vi "12_Eoff.vi"(0 "file path (IN)":path, 1 "VGE":dbl, 5 "Project #":string, 7 "Request #":string, 9 "TEST #":string, 11 "error in (no error)":errorcluster) -> (4 "file path (OUT)":path, 6 "Eoff (uj)":dbl, 8 "DONE Eoff":bool, 10 "OFF Region":waveform(dbl)[](graph) caption="Eoff (uj)", 15 "error out":errorcluster)   [LabVIEW 2020]
uses:
  <vilib>/Waveform/WDTOps.llb/WDT Waveform Duration DBL.vi
  <vilib>/Waveform/WDTOps.llb/WDT Get Waveform Subset DBL.vi
  <vilib>/measure/mamon.llb/Trigger Detection for 1 Channel.vi
  <vilib>/measure/mascope.llb/Transition Measurements 1 chan.vi
  <vilib>/measure/NI_MAPro.lvlib
panel:
  in  "Decision ?":bool
  out "Cursor a : Channel 2":dbl
  in  "Cursor a : Channel 2\nfall edge tolerance":dbl=0.1
  in  "Cursor a : Channel 2\nfall edge number":i32=1 min=1
  out "Eoff : XY Graph":cluster{"X":dbl, "Y":dbl}[](graph)
  out "Eoff Area Y-axis":dbl[](array[numeric])
  out "Eoff Area X-axis":dbl[](array[numeric])
  out "90% Vge":dbl
  out "measurement info (CH2)":T1 {"ref levels"."ref units" items=["absolute", "relative"]; "ref levels"."high ref level" format="%.2p"; "ref levels"."low ref level" format="%.2p"; "ref levels"."mid ref level" format="%.2p"; "end time" format="%.6e"; "start time" format="%.6e"}
  in  "reference  levels (CH2 initialize)":T2={"high ref level"=90.0, "mid ref level"=50.0, "low ref level"=10.0, "ref units"=1} {"ref units" items=["absolute", "percent"]; "high ref level" format="%0.2f"; "low ref level" format="%0.2f"; "mid ref level" format="%0.2f"}
  out "Waveform Graph":waveform(dbl)[](graph)
  # "From 90% Vge to Most Right of Screen"
  # "Default = 1"
  # "Default = 0.1"
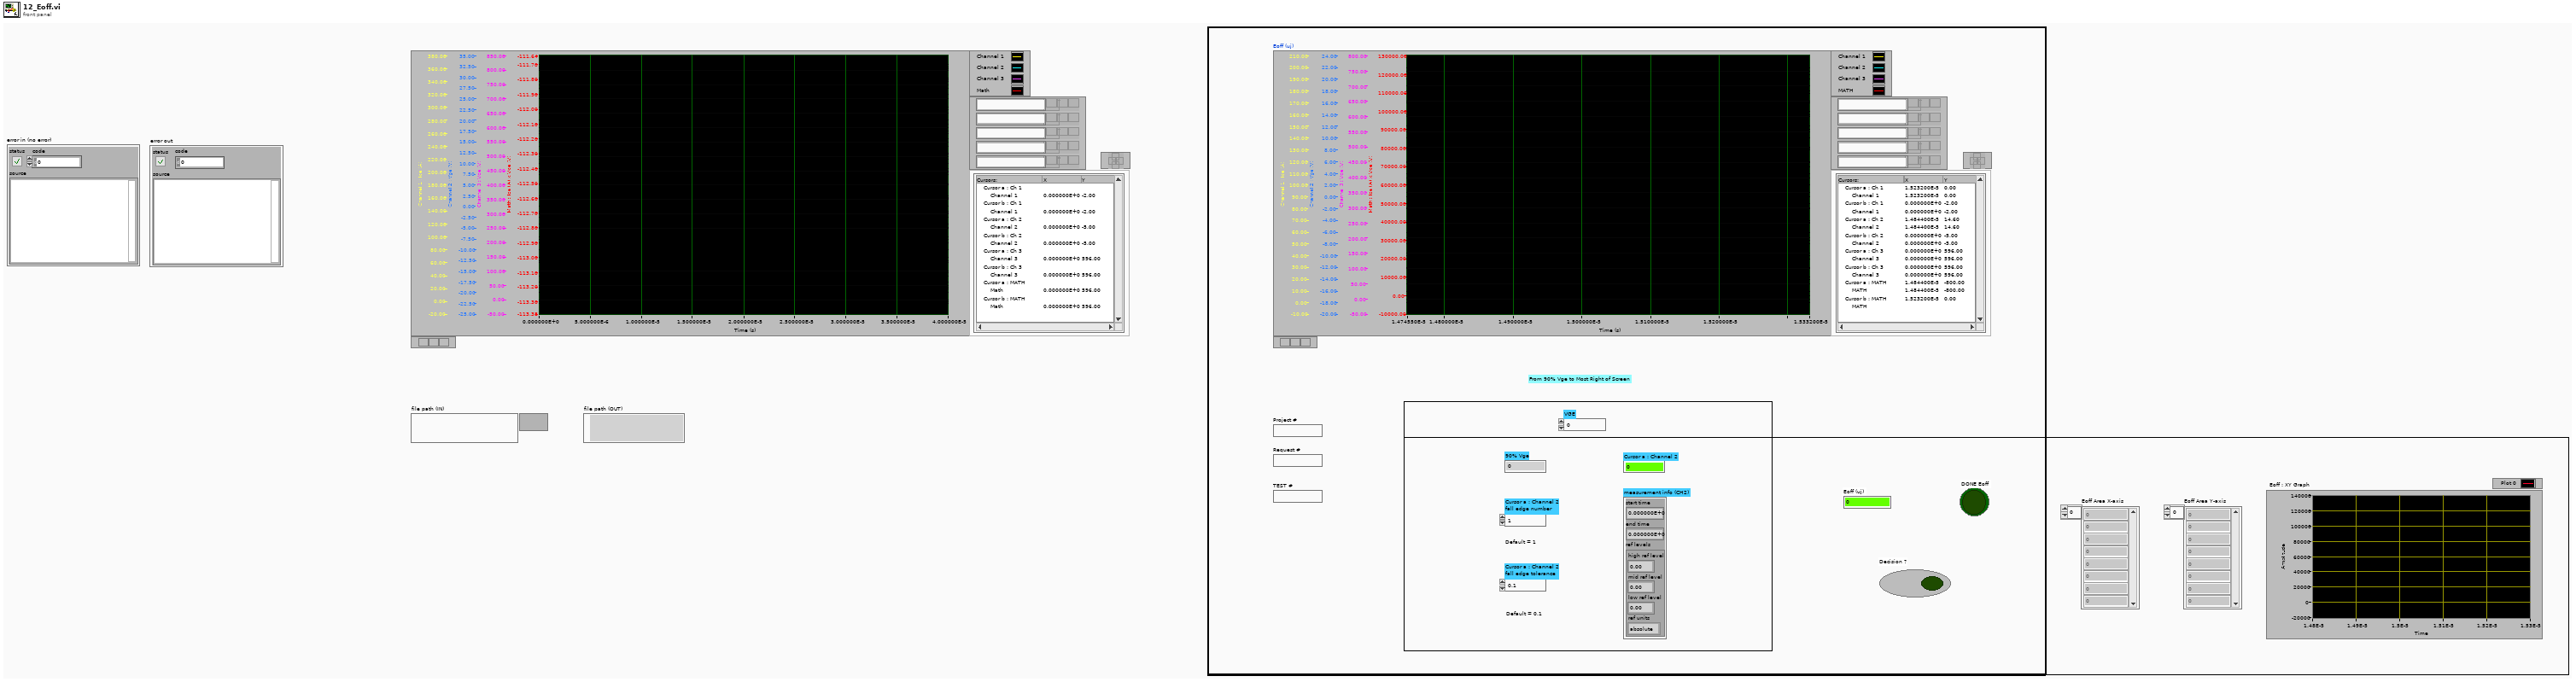
[diagram p1: front panel]
types:
  T1 = cluster{"start time":dbl, "end time":dbl, "ref levels":cluster{"high ref level":dbl, "mid ref level":dbl, "low ref level":dbl, "ref units":u16}}
  T2 = cluster{"high ref level":dbl, "mid ref level":dbl, "low ref level":dbl, "ref units":u16}
  T3 = enum32{"Invalid", "Standard", "Closed", "Hidden", "Minimized", "Maximized"}
  T4 = typedef "imagedata.ctl" = cluster{"image type":i32, "image depth":i32, "image":u8[], "mask":u8[], "colors":u32[], "Rectangle":cluster{"left":i16, "top":i16, "right":i16, "bottom":i16}}
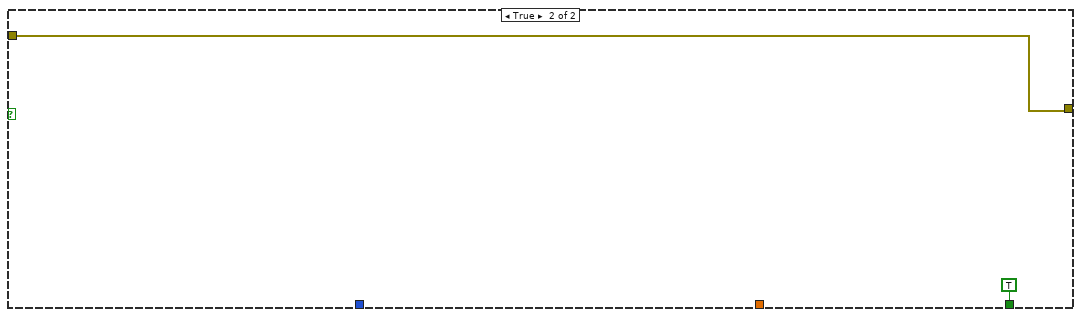
[diagram p8: hidden frame]
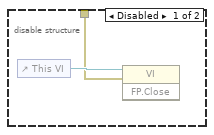
[diagram p9: hidden frame]
diagram:
  w10 = 0.0 ("Eoff (uj)")
  w14 = errorcluster {"status"=FALSE, "code"=0, "source"=""} ("error out")
  w3 = FALSE ("DONE Tdon")
  w15 = waveform(dbl)[] [] ("Waveform Graph")
  n1 = local write "error out"(w14) -> ()
  n2 = local write "error in (no error)"(w14) -> ()
  n3 = local write "Cursor a : Channel 2\nfall edge tolerance"(0.1 ("Cursor a : Channel 2\nfall edge tolerance")) -> ()
  n4 = local write "Cursor a : Channel 2\nfall edge number"(1 ("Cursor a : Channel 2\nfall edge number")) -> ()
  n5 = local write "DONE Eoff"(w3) -> ()
  n6 = local write "Decision ?"(w3) -> ()
  n7 = local write "Eoff (uj)"(w10) -> ()
  n8 = local write "Cursor a : Channel 2"(w10) -> ()
  n9 = local write "Waveform Graph"(w15) -> ()
  n10 = local write "OFF Region"(w15) -> ()
  n11 = flat-sequence {
    tunnel: [w17] -> w5
    tunnel: ["file path (IN)"] -> w4
    tunnel: [w27] -> w9
    tunnel: [w26] -> w7
    tunnel: w5 -> [w25]
    tunnel: w4 -> [w24]
    tunnel: w9 -> [w376]
    tunnel: [w375] -> w8
    tunnel: w7 -> [w374]
    tunnel: [w374] -> w6
    tunnel: w8 -> [w389]
    tunnel: w6 -> [w390]
    frame #0 {
      n12 = control-ref of="This VI"() -> (w19:refnum<vi>)
      n13 = invoke class="VI" method="FP.Open"(reference=w19, error in="error in (no error)", "Activate"=TRUE ("Activate?"), "State"=T3."Maximized") -> (error out=w20:errorcluster)  [unwired: 1 in, 4 out]
      n14 = property class="VI"(reference=w19, error in=w20, "Front Panel.Closeable"=TRUE ("Front Panel Window:Closeable")) -> (error out=w17:errorcluster)  [unwired: 1 out]
    }
    frame #1 {
      n15 = while {
        shift-right: [w33] -> w27
        shift-left: w25 -> [w35]
        tunnel: [w30] -> w26
        tunnel: w24 -> [w29]
        stop <- w31 stop-if-true
        n16 = flat-sequence {
          tunnel: [w70] -> w62
          tunnel: w35 -> [w76]
          tunnel: [w76] -> w34
          tunnel: w29 -> [w70]
          tunnel: w62 -> [w178]
          tunnel: [w110] -> w61
          tunnel: [w109] -> w60
          tunnel: [w99] -> w59
          tunnel: [w81] -> w58
          tunnel: [w79] -> w57
          tunnel: w34 -> [w183]
          tunnel: [w77] -> w28
          tunnel: w61 -> [w208]
          tunnel: w60 -> [w201]
          tunnel: [w213] -> w56
          tunnel: w59 -> [w212]
          tunnel: [w212] -> w55
          tunnel: [w199] -> w54
          tunnel: [w205] -> w53
          tunnel: w58 -> [w209]
          tunnel: [w209] -> w52
          tunnel: w57 -> [w206]
          tunnel: w28 -> [w200]
          tunnel: w56 -> [w250]
          tunnel: [w249] -> w51
          tunnel: w55 -> [w255]
          tunnel: [w255] -> w50
          tunnel: w54 -> [w254]
          tunnel: [w254] -> w49
          tunnel: w53 -> [w253]
          tunnel: [w253] -> w48
          tunnel: w52 -> [w252]
          tunnel: [w252] -> w47
          tunnel: w51 -> [w266]
          tunnel: [w257] -> w46
          tunnel: w50 -> [w267]
          tunnel: [w267] -> w45
          tunnel: w49 -> [w265]
          tunnel: [w265] -> w44
          tunnel: w48 -> [w264]
          tunnel: [w264] -> w43
          tunnel: w47 -> [w262]
          tunnel: w46 -> [w348]
          tunnel: [w347] -> w42
          tunnel: w45 -> [w355]
          tunnel: [w355] -> w41
          tunnel: w44 -> [w344]
          tunnel: w43 -> [w343]
          tunnel: [w343] -> w40
          tunnel: [w344] -> w39
          tunnel: w42 -> [w365]
          tunnel: [w366] -> w38
          tunnel: w41 -> [w367]
          tunnel: [w367] -> w37
          tunnel: w40 -> [w360]
          tunnel: w39 -> [w359]
          tunnel: w38 -> [w370]
          tunnel: w37 -> [w368]
          tunnel: [w369] -> w36
          tunnel: [w368] -> w30
          frame #0 {
            w69 = FALSE ("DONE Tdon")
            w75 = waveform(dbl)[] [] ("Waveform Graph")
            w74 = 0.0 ("Eoff (uj)")
            n17 = local write "DONE Eoff"(w69) -> ()
            n18 = local write "Decision ?"(w69) -> ()
            n19 = local write "Eoff (uj)"(w74) -> ()
            n20 = local write "Cursor a : Channel 2"(w74) -> ()
            n21 = local write "Waveform Graph"(w75) -> ()
            n22 = local write "OFF Region"(w75) -> ()
            n23 = local write "Eoff Area Y-axis"(dbl[] [] ("Eoff Area X-axis")) -> ()
            n24 = local write "Eoff Area X-axis"(dbl[] [] ("Eoff Area Y-axis")) -> ()
            n25 = local write "Eoff : XY Graph"(cluster{"X":dbl, "Y":dbl}[] [] ("Eoff : XY Graph")) -> ()
          }
          frame #1 {
            w78 = 0.0 ("start samples/time")
            w88 = u16 1 items=["Samples", "Relative Time"] ("start/duration format")
            w160 = u16 1 items=["Samples", "Relative Time"] ("start/duration format")
            w170 = u16 1 items=["Samples", "Relative Time"] ("start/duration format")
            w171 = u16 1 items=["Samples", "Relative Time"] ("start/duration format")
            # "Channel 3"
            # "Channel 1"
            # "Channel MATH"
            # "MATH = Ch1 x Ch3"
            # "Channel 1"
            # "Channel 3"
            # "Channel 2"
            # "dt"
            # "Ch2"
            # "Ch1"
            n26 = call "3_ReadDatatoWaveform.vi"("error in (no error)"=w183, "file path (IN)"=w178) -> ("error out"=w157:errorcluster, "Waveform Graph"=→"Waveform Graph":waveform(dbl)[], "file path (OUT)"=w99:path, "dt"=w179:dbl, "Ch 2 Data"=w176:dbl[], "Ch 3 Data"=w180:dbl[], "Ch 1 Data"=w177:dbl[])  [unwired: 3 in]
            n27 = call <vilib>:"Beep.vi"("use system alert? (T)"=FALSE, "duration (msec)"=u32 200, "frequency (Hz)"=u32 2000) -> ()  [unwired: 9 in]
            n28 = To Time Stamp(1:0.0 ("number")) -> (0:w181:timestamp)
            n29 = disable-structure shown="Enabled" {
              disable-tunnel: w181 -> [w198 _]
              disable-tunnel: w179 -> [w197 _]
              disable-tunnel: w180 -> [w196 _]
              disable-tunnel: [w195 _] -> w95
              frame Enabled {
                # "Channel 3"
                n30 = Bundle By Name("Y"=w196, "dt"=w197, "t0"=w198) -> (w195:waveform(dbl))  [unwired: 1 in]
              }
              frame Disabled {
              }
            }
            n31 = disable-structure shown="Enabled" {
              disable-tunnel: w181 -> [w194 _]
              disable-tunnel: w179 -> [w193 _]
              disable-tunnel: w176 -> [w192 _]
              disable-tunnel: [w191 _] -> w159
              frame Enabled {
                # "Channel 2"
                n32 = Bundle By Name("Y"=w192, "dt"=w193, "t0"=w194) -> (w191:waveform(dbl))  [unwired: 1 in]
              }
              frame Disabled {
              }
            }
            n33 = disable-structure shown="Enabled" {
              disable-tunnel: w181 -> [w190 _]
              disable-tunnel: w179 -> [w189 _]
              disable-tunnel: w177 -> [w188 _]
              disable-tunnel: [w187 _] -> w96
              frame Enabled {
                # "Channel 1"
                n34 = Bundle By Name("Y"=w188, "dt"=w189, "t0"=w190) -> (w187:waveform(dbl))  [unwired: 1 in]
              }
              frame Disabled {
              }
            }
            n35 = Unbundle By Name(w95) -> ("Y"=w92:dbl[])
            n36 = Unbundle By Name(w96) -> ("Y"=w93:dbl[], "dt"=w80:dbl, "t0"=w94:timestamp)
            n37 = for {
              tunnel: w93 -> [w186] mode=indexing
              tunnel: w92 -> [w185] mode=indexing
              tunnel: [w184] -> w91 mode=indexing
              n38 = Multiply(x=w186, y=w185) -> (x*y=w184:dbl)
            }
            n39 = Bundle By Name("Y"=w91, "dt"=w80, "t0"=w94) -> (w83:waveform(dbl))  [unwired: 1 in]
            n40 = call-poly <vilib>:"Waveform Duration.vi"("waveform in"=w83) -> ("error out"=w84:errorcluster, "duration"=w86:dbl, "waveform out"=w89:waveform(dbl))  [unwired: 8 in]
            n41 = call-poly <vilib>:"Waveform Duration.vi"("error in (no error)"=w157, "waveform in"=w95) -> ("error out"=w164:errorcluster, "duration"=w162:dbl, "waveform out"=w97:waveform(dbl))  [unwired: 7 in]
            n42 = call-poly <vilib>:"Waveform Duration.vi"("error in (no error)"=w157, "waveform in"=w159) -> ("error out"=w165:errorcluster, "duration"=w168:dbl, "waveform out"=w166:waveform(dbl))  [unwired: 7 in]
            n43 = call-poly <vilib>:"Waveform Duration.vi"("error in (no error)"=w157, "waveform in"=w96) -> ("error out"=w175:errorcluster, "duration"=w172:dbl, "waveform out"=w174:waveform(dbl))  [unwired: 7 in]
            n44 = Divide(x=w86, y=2.0) -> (x/y=w87:dbl)
            n45 = Divide(x=w162, y=2.0) -> (x/y=w161:dbl)
            n46 = Divide(x=w168, y=2.0) -> (x/y=w169:dbl)
            n47 = Divide(x=w172, y=2.0) -> (x/y=w79:dbl)
            n48 = call-poly <vilib>:"Get Waveform Subset.vi"("start/duration format"=w160, "error in (no error)"=w164, "duration"=w161, "start samples/time"=w78, "waveform in"=w97) -> ("error out"=w154:errorcluster, "waveform out"=w98:waveform(dbl))  [unwired: 1 in, 2 out]
            n49 = call-poly <vilib>:"Get Waveform Subset.vi"("start/duration format"=w88, "error in (no error)"=w84, "duration"=w87, "start samples/time"=w78, "waveform in"=w89) -> ("error out"=w82:errorcluster, "waveform out"=w81:waveform(dbl))  [unwired: 1 in, 2 out]
            n50 = call-poly <vilib>:"Get Waveform Subset.vi"("start/duration format"=w170, "error in (no error)"=w165, "duration"=w169, "start samples/time"=w78, "waveform in"=w166) -> ("error out"=w155:errorcluster, "waveform out"=w110:waveform(dbl))  [unwired: 1 in, 2 out]
            n51 = call-poly <vilib>:"Get Waveform Subset.vi"("start/duration format"=w171, "error in (no error)"=w175, "duration"=w79, "start samples/time"=w78, "waveform in"=w174) -> ("error out"=w156:errorcluster, "waveform out"=w77:waveform(dbl))  [unwired: 1 in, 2 out]
            n52 = Build Array(w77, w110, w98, w81) -> (→"OFF Region":waveform(dbl)[])
            n53 = Merge Errors(w156, w155, w154, w82) -> (w107:errorcluster)
            n54 = property on="OFF Region" class="WFGraph (strict)"(error in=w107) -> (error out=w106:errorcluster, "Width"=w105:u32)  [unwired: 1 in, 1 out]
            n55 = property on="OFF Region" class="WFGraph (strict)"(error in=w106, "Caption.Justify"=enum16{"Left", "Center", "Right"}."Left" ("Caption.Justification"), "Caption.Width"=w105, "Caption.FontBold"=TRUE ("Caption.Font:Bold"), "Caption.FontColor"=u32 16860 ("Caption.Font:Color"), "Caption.FontSize"=u32 24 ("Caption.Font:Size"), "Caption.Text"="Eoff (uj)") -> (error out=w101:errorcluster)  [unwired: 1 in, 1 out]
            n56 = property on="OFF Region" class="WFGraph (strict)"(error in=w101, "XScale.Offset"=w78) -> (error out=w134:errorcluster)  [unwired: 1 in, 1 out]
            n57 = property on="OFF Region" class="WFGraph (strict)"(error in=w134, "Active Cursor"=u32 0, "Cursor.Cursor X"=0.0 ("Cursor.Cursor Position:Cursor X"), "Cursor.Cursor Y"=0.0 ("Cursor.Cursor Position:Cursor Y"), "Cursor.Visible"=FALSE) -> (error out=w133:errorcluster)  [unwired: 1 in, 1 out]
            n58 = property on="OFF Region" class="WFGraph (strict)"(error in=w133, "Active Cursor"=u32 1, "Cursor.Cursor X"=0.0 ("Cursor.Cursor Position:Cursor X"), "Cursor.Cursor Y"=0.0 ("Cursor.Cursor Position:Cursor Y"), "Cursor.Visible"=FALSE) -> (error out=w132:errorcluster)  [unwired: 1 in, 1 out]
            n59 = property on="OFF Region" class="WFGraph (strict)"(error in=w132, "Active Cursor"=u32 2, "Cursor.Cursor X"=0.0 ("Cursor.Cursor Position:Cursor X"), "Cursor.Cursor Y"=0.0 ("Cursor.Cursor Position:Cursor Y"), "Cursor.Visible"=FALSE) -> (error out=w131:errorcluster)  [unwired: 1 in, 1 out]
            n60 = property on="OFF Region" class="WFGraph (strict)"(error in=w131, "Active Cursor"=u32 3, "Cursor.Cursor X"=0.0 ("Cursor.Cursor Position:Cursor X"), "Cursor.Cursor Y"=0.0 ("Cursor.Cursor Position:Cursor Y"), "Cursor.Visible"=FALSE) -> (error out=w114:errorcluster)  [unwired: 1 in, 1 out]
            n61 = property on="OFF Region" class="WFGraph (strict)"(error in=w114, "Active Cursor"=u32 4, "Cursor.Cursor X"=0.0 ("Cursor.Cursor Position:Cursor X"), "Cursor.Cursor Y"=0.0 ("Cursor.Cursor Position:Cursor Y"), "Cursor.Visible"=FALSE) -> (error out=w113:errorcluster)  [unwired: 1 in, 1 out]
            n62 = property on="OFF Region" class="WFGraph (strict)"(error in=w113, "Active Cursor"=u32 5, "Cursor.Cursor X"=0.0 ("Cursor.Cursor Position:Cursor X"), "Cursor.Cursor Y"=0.0 ("Cursor.Cursor Position:Cursor Y"), "Cursor.Visible"=FALSE) -> (error out=w112:errorcluster)  [unwired: 1 in, 1 out]
            n63 = property on="OFF Region" class="WFGraph (strict)"(error in=w112, "Active Cursor"=u32 6, "Cursor.Cursor X"=0.0 ("Cursor.Cursor Position:Cursor X"), "Cursor.Cursor Y"=0.0 ("Cursor.Cursor Position:Cursor Y"), "Cursor.Visible"=FALSE) -> (error out=w111:errorcluster)  [unwired: 1 in, 1 out]
            n64 = property on="OFF Region" class="WFGraph (strict)"(error in=w111, "Active Cursor"=u32 7, "Cursor.Cursor X"=0.0 ("Cursor.Cursor Position:Cursor X"), "Cursor.Cursor Y"=0.0 ("Cursor.Cursor Position:Cursor Y"), "Cursor.Visible"=FALSE) -> (error out=w109:errorcluster)  [unwired: 1 in, 1 out]
          }
          frame #2 {
            w230 = u16 0 items=["falling", "rising"] ("polarity (rising)")
            # "Cursor a : Channel 1"
            # "Channel 1"
            # "2nd PARAMETER"
            # "MOST RIGHT SCREEN"
            # "Cursor a : Channel 2"
            # "End Time 1st Cursor"
            # "2nd PARAMETER"
            # "MOST RIGHT SCREEN"
            # "1st PARAMETER"
            # "Channel 2"
            n65 = Divide(x=90.0, y=100.0) -> (x/y=w234:dbl)
            n66 = Multiply(x=w234, y="VGE") -> (x*y=w207:dbl)
            "90% Vge" <- w207
            n67 = Add(x=w207, y="Cursor a : Channel 2\nfall edge tolerance") -> (x+y=w229:dbl)
            n68 = Subtract(x=w207, y="Cursor a : Channel 2\nfall edge tolerance") -> (x-y=w228:dbl)
            n69 = Bundle By Name(cluster="reference  levels (CH2 initialize)", "high ref level"=w229, "mid ref level"=w207, "low ref level"=w228, "ref units"=u16 0) -> (w225:T2)
            n70 = call-poly <vilib>:"Transition Measurements.vi"("edge number (1)"="Cursor a : Channel 2\nfall edge number", "error in (no error)"=w201, "reference levels"=w225, "polarity (rising)"=w230, "signal in"=w208) -> ("error out"=w219:errorcluster, "measurement info"=w224:T1)  [unwired: 1 in, 4 out]
            "measurement info (CH2)" <- w224
            n71 = disable-structure shown="Enabled" {
              disable-tunnel: [w245 _] -> w202
              disable-tunnel: w201 -> [w244 _]
              disable-tunnel: w200 -> [w243 _]
              disable-tunnel: [w241 _] -> w199
              frame Enabled {
                w247 = u16 0 items=["Falling Edge", "Rising Edge"] ("trigger slope")
                w246 = u16 1 items=["Index", "Time"] ("location mode")
                n72 = call-poly <vilib>:"Basic Level Trigger Detection.vi"("signal in"=w243, "level"=0.2, "hysteresis"=10.0, "location mode"=w246, "error in (no error)"=w244, "trigger slope"=w247) -> ("trigger location"=w241:dbl, "error out"=w245:errorcluster)  [unwired: 7 in, 1 out]
              }
              frame Disabled {
              }
            }
            n73 = Unbundle By Name(w224) -> ("end time"=w205:dbl)
            n74 = call <vilib>:"Beep.vi"("use system alert? (T)"=FALSE, "duration (msec)"=u32 200, "frequency (Hz)"=u32 2000) -> ()  [unwired: 9 in]
            n75 = disable-structure shown="Disabled" {
              disable-tunnel: w206 -> [w237 _]
              disable-tunnel: [w236 _] -> _
              disable-tunnel: w205 -> [w235 _]
              frame Disabled {
                n76 = Add(x=w237, y=w235) -> (x+y=w239:dbl)
                n77 = Divide(x=w239, y=2.0) -> (x/y=w236:dbl)
              }
              frame Enabled {
              }
            }
            n78 = disable-structure shown="Disabled" {
              frame Disabled {
                # "3"
                # "Cursor b : Channel 2"
              }
              frame Enabled {
              }
            }
            n79 = property on="OFF Region" class="WFGraph (strict)"(error in=w219, "Active Cursor"=u32 2, "Cursor.Cursor X"=w205, "Cursor.Visible"=TRUE, "Cursor.Cursor Name Visible"=TRUE) -> (error out=w214:errorcluster)  [unwired: 1 in, 1 out]
            n80 = property on="OFF Region" class="WFGraph (strict)"(error in=w202, "Active Cursor"=u32 0, "Cursor.Cursor X"=w199, "Cursor.Visible"=TRUE, "Cursor.Cursor Name Visible"=TRUE) -> (error out=w215:errorcluster)  [unwired: 1 in, 1 out]
            n81 = Merge Errors(w215, w214) -> (w213:errorcluster)
          }
          frame #3 {
            # "Cursor a : Channel 2"
            n82 = property on="OFF Region" class="WFGraph (strict)"(error in=w250, "Active Cursor"=u32 2) -> (error out=w249:errorcluster, "Cursor.Cursor Y"=→"Cursor a : Channel 2":dbl)  [unwired: 1 in, 1 out]
          }
          frame #4 {
            n83 = flat-sequence {
              tunnel: w266 -> [w271]
              tunnel: w265 -> [w273]
              tunnel: w264 -> [w272]
              tunnel: [w268] -> w263
              tunnel: w263 -> [w282]
              tunnel: w261 -> [w281]
              tunnel: [w280] -> w260
              tunnel: w260 -> [w323]
              tunnel: [w325] -> w259
              tunnel: [w324] -> w258
              tunnel: [w323] -> w256
              tunnel: w259 -> [w331]
              tunnel: w258 -> [w330]
              tunnel: [w329] -> w257
              tunnel: w256 -> [w329]
              frame #0 {
                # "Cursor a : MATH"
                # "Cursor b : MATH"
                n84 = property on="OFF Region" class="WFGraph (strict)"(error in=w271, "Active Cursor"=u32 7, "Cursor.Cursor X"=w273, "Cursor.Visible"=TRUE, "Cursor.Cursor Name Visible"=TRUE) -> (error out=w269:errorcluster)  [unwired: 1 in, 1 out]
                n85 = property on="OFF Region" class="WFGraph (strict)"(error in=w271, "Active Cursor"=u32 6, "Cursor.Cursor X"=w272, "Cursor.Visible"=TRUE, "Cursor.Cursor Name Visible"=TRUE) -> (error out=w270:errorcluster)  [unwired: 1 in, 1 out]
                n86 = Merge Errors(w269, w270) -> (w268:errorcluster)
              }
              frame #1 {
                n87 = while {
                  tunnel: w282 -> [w290]
                  tunnel: w281 -> [w284]
                  tunnel: [w283] -> w280
                  i -> [w285]
                  stop <- w288 stop-if-true
                  # "Cursor b : MATH"
                  # "Cursor a : MATH"
                  n88 = property on="OFF Region" class="WFGraph (strict)"(error in=w290, "Active Cursor"=u32 7) -> (error out=w294:errorcluster, "Cursor.Cursor X"=w296:dbl)  [unwired: 1 in, 1 out]
                  n89 = property on="OFF Region" class="WFGraph (strict)"(error in=w290, "Active Cursor"=u32 6) -> (error out=w293:errorcluster, "Cursor.Cursor X"=w295:dbl)  [unwired: 1 in, 1 out]
                  n90 = Merge Errors(w293, w294) -> (w286:errorcluster)
                  n91 = Equal?(x=w295, y=w296) -> (x = y?=w289:bool)
                  n92 = case shown="False" w289 {
                    tunnel: [FALSE TRUE] -> w288
                    tunnel: w286 -> [w301 w321]
                    tunnel: w285 -> [w300 _]
                    tunnel: w284 -> [w298 _]
                    tunnel: [w297 w321] -> w283
                    frame False {
                      n93 = flat-sequence {
                        tunnel: w301 -> [w311]
                        tunnel: w300 -> [w306]
                        tunnel: [w303] -> w299
                        tunnel: w299 -> [w316]
                        tunnel: w298 -> [w314]
                        tunnel: [w313] -> w297
                        frame #0 {
                          # "Cursor a : MATH"
                          n94 = property on="OFF Region" class="WFGraph (strict)"(error in=w311, "Active Cursor"=u32 6) -> (error out=w303:errorcluster, "Cursor.Cursor X"=w308:dbl, "Cursor.Cursor Y"=w307:dbl)  [unwired: 1 in, 1 out]
                          n95 = local read "Eoff Area Y-axis"() -> (w309:dbl[])
                          n96 = local read "Eoff Area X-axis"() -> (w310:dbl[])
                          n97 = Insert Into Array(array=w309, index=w306, new element=w307) -> (w304:dbl[])
                          n98 = Insert Into Array(array=w310, index=w306, new element=w308) -> (w305:dbl[])
                          n99 = local write "Eoff Area X-axis"(w305) -> ()
                          n100 = local write "Eoff Area Y-axis"(w304) -> ()
                        }
                        frame #1 {
                          # "Cursor a : MATH"
                          # "Cursor a : MATH"
                          n101 = property on="OFF Region" class="WFGraph (strict)"(error in=w316, "Active Cursor"=u32 6) -> (error out=w315:errorcluster, "Cursor.Cursor X"=w318:dbl)  [unwired: 1 in, 1 out]
                          n102 = Add(x=w318, y=w314) -> (x+y=w317:dbl)
                          n103 = property on="OFF Region" class="WFGraph (strict)"(error in=w315, "Active Cursor"=u32 6, "Cursor.Cursor X"=w317) -> (error out=w313:errorcluster)  [unwired: 1 in, 1 out]
                        }
                      }
                    }
                    frame True {
                    }
                  }
                  n104 = Wait (ms)(milliseconds to wait=u32 1) -> ()  [unwired: 1 out]
                }
              }
              frame #2 {
                n105 = local read "Eoff Area X-axis"() -> (w325:dbl[])
                n106 = local read "Eoff Area Y-axis"() -> (w324:dbl[])
                n107 = Build Cluster Array(w325, w324) -> (w326:cluster{dbl, dbl}[])
                n108 = local write "Eoff : XY Graph"(w326) -> ()
                n109 = Wait (ms)(milliseconds to wait=u32 50) -> ()  [unwired: 1 out]
              }
              frame #3 {
                n110 = Wait (ms)(milliseconds to wait=u32 50) -> ()  [unwired: 1 out]
                n111 = Delete From Array(array=w331, index=0) -> (array with subset deleted=w341:dbl[])  [unwired: 1 in, 1 out]
                n112 = Delete From Array(array=w330, index=0) -> (array with subset deleted=w335:dbl[])  [unwired: 1 in, 1 out]
                n113 = Subtract(x=w341, y=w331) -> (x-y=w340:dbl[])
                n114 = Add(x=w335, y=w330) -> (x+y=w339:dbl[])
                n115 = Compound Arithmetic op=MULTIPLY(w340, w339, invert 2.0 ("Numeric")) -> (w337:dbl[])
                n116 = Add Array Elements(numeric array=w337) -> (sum=w333:dbl)
                n117 = Multiply(x=w333, y=1000000.0) -> (x*y=→"Eoff (uj)":dbl)
              }
            }
            n118 = Unbundle By Name(w262) -> ("dt"=w261:dbl)
          }
          frame #5 {
            # "Cursor a : MATH"
            # "Cursor b : MATH"
            n119 = property on="OFF Region" class="WFGraph (strict)"(error in=w348, "Active Cursor"=u32 7, "Cursor.Cursor X"=w344, "Cursor.Visible"=TRUE, "Cursor.Cursor Name Visible"=TRUE) -> (error out=w345:errorcluster)  [unwired: 1 in, 1 out]
            n120 = property on="OFF Region" class="WFGraph (strict)"(error in=w348, "Active Cursor"=u32 6, "Cursor.Cursor X"=w343, "Cursor.Visible"=TRUE, "Cursor.Cursor Name Visible"=TRUE) -> (error out=w346:errorcluster)  [unwired: 1 in, 1 out]
            n121 = Merge Errors(w345, w346) -> (w347:errorcluster)
          }
          frame #6 {
            # "2nd Cursor"
            # "1st Cursor"
            n122 = Subtract(x=w360, y=1e-07) -> (x-y=w361:dbl)
            n123 = Add(x=w359, y=1e-07) -> (x+y=w362:dbl)
            n124 = call <vilib>:"Beep.vi"("use system alert? (T)"=FALSE, "duration (msec)"=u32 200, "frequency (Hz)"=u32 2000) -> ()  [unwired: 9 in]
            n125 = property on="OFF Region" class="WFGraph (strict)"(error in=w365, "XScale.Minimum"=w361, "XScale.Maximum"=w362) -> (error out=w366:errorcluster)  [unwired: 1 in, 1 out]
          }
          frame #7 {
            n126 = while {
              shift-right: [w371] -> w369
              shift-left: w370 -> [w371]
              stop <- "Decision ?" stop-if-true
              n127 = Wait (ms)(milliseconds to wait=u32 100) -> ()  [unwired: 1 out]
            }
          }
        }
        n128 = while {
          tunnel: [w64] -> w31
          shift-right: [w67] -> w33
          shift-left: w36 -> [w68]
          stop <- w66 stop-if-true
          n129 = Wait (ms)(milliseconds to wait=u32 100) -> ()  [unwired: 1 out]
          n130 = call "Display Message to User"("error in (no error)"=w68) -> ("error out"=w67:errorcluster, "NO"=w64:bool)  [unwired: 9 in]
          n131 = Or(x=w64, y=TRUE) -> (x .or. y?=w66:bool)
        }
        n132 = Wait (ms)(milliseconds to wait=u32 100) -> ()  [unwired: 1 out]
      }
    }
    frame #2 {
      w380 = "_"
      n133 = invoke on="OFF Region" class="WFGraph (strict)" method="Get Image"(error in=w376) -> (error out=w382:errorcluster, "image data"=w385:T4)  [unwired: 5 in, 4 out]
      n134 = Concatenate Strings("C:\\Inductive_Switching_Project\\IndSw_Image\\" ("string"), "Project #", w380, "Request #", w380, "TEST #", w380, "Eoff" ("string"), ".png" ("string")) -> (w386:string)
      n135 = String To Path(string=w386) -> (path=w384:path)
      n136 = call <vilib>:"Write PNG File.vi"("error in (no error)"=w382, "image data"=w385, "path to PNG file"=w384) -> ("error out"=w375:errorcluster)  [unwired: 7 in, 1 out]
      "DONE Eoff" <- TRUE ("DONE Tdon")
    }
    frame #3 {
      n137 = disable-structure shown="Enabled" {
        disable-tunnel: w389 -> [w391 _]
        frame Disabled {
          n138 = control-ref of="This VI"() -> (w392:refnum<vi>)
          n139 = invoke class="VI" method="FP.Close"(reference=w392, error in=w391) -> ()  [unwired: 1 in, 3 out]
        }
        frame Enabled {
        }
      }
      "error out" <- w389
      "file path (OUT)" <- w390
    }
  }
  "Eoff : XY Graph" <- cluster{"X":dbl, "Y":dbl}[] [] ("Eoff : XY Graph")
  "Eoff Area X-axis" <- dbl[] [] ("Eoff Area X-axis")
  "Eoff Area Y-axis" <- dbl[] [] ("Eoff Area Y-axis")
